vi "ReadMaxCtrlV.vi"(8 "error in (no error)":errorcluster, 11 "APDClass in":refnum<class "APDClass.lvclass">) -> (0 "error out":errorcluster, 2 "Numeric":dbl, 3 "APDClass out":refnum<class "APDClass.lvclass">)   [LabVIEW 2020, in "APDClass.lvclass"]
uses:
  APDClass.lvclass
  APDClass.lvclass/APDClass.ctl
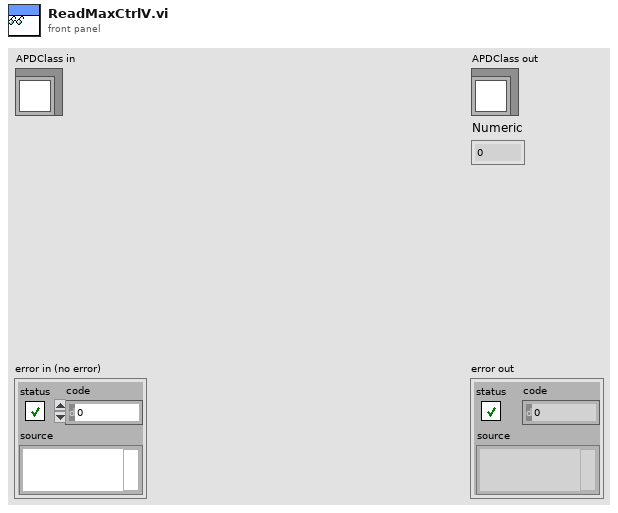
[diagram p1: front panel]
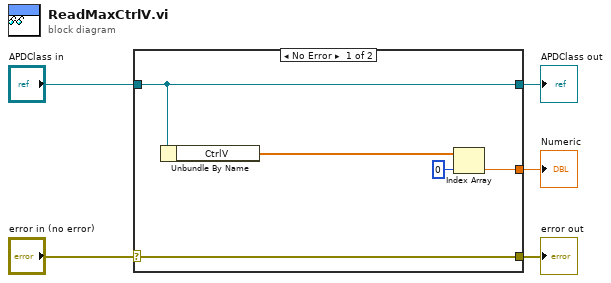
[diagram p0: block diagram]
diagram:
  n1 = case shown="No Error" "error in (no error)" {
    selector: "error in (no error)" -> [w10 w11]
    tunnel: [w10 w11] -> w4
    tunnel: [w9 w12] -> w2
    tunnel: "APDClass in" -> [w9 w12]
    tunnel: [w7 _] -> w1
    frame No Error {
      n2 = Unbundle By Name(w9) -> ("CtrlV"=w8:dbl[])
      n3 = Index Array(array=w8, index=0) -> (element=w7:dbl)
    }
    frame Error {
    }
  }
  "error out" <- w4
  "APDClass out" <- w2
  "Numeric" <- w1
